vi "SVFA Get Spectrum Value.vi"   [LabVIEW 2017]
doc: "Extracts the value of the spectrum at the specified frequency. Use the frequency coercion control to specify how the frequency should be coerced if it does not exactly coincide with a frequency line. This VI operates on any real-valued spectrum. Wire data to the <B>spectrum</B> input to determine the polymorphic instance to use or manually select the instance."
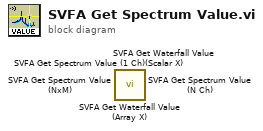
[diagram p0: block diagram]
diagram:
  n1 = call <vilib>:"SVFA Get Waterfall Value (Array X).vi"() -> ()  [unwired: 18 in, 2 out]
  n2 = call <vilib>:"SVFA Get Waterfall Value (Scalar X).vi"() -> ()  [unwired: 18 in, 2 out]
  n3 = call <vilib>:"SVFA Get Spectrum Value (NxM).vi"() -> ()  [unwired: 15 in, 5 out]
  n4 = call <vilib>:"SVFA Get Spectrum Value (N Ch).vi"() -> ()  [unwired: 15 in, 5 out]
  n5 = call <vilib>:"SVFA Get Spectrum Value (1 Ch).vi"() -> ()  [unwired: 15 in, 5 out]
